vi "DAQ_Dyn Dig Gen Initialize.vi"(0 "Physical Channels":tag, 7 "Global Channels":refnum<k21>, 11 "error in":errorcluster) -> (4 "DAQmx Task Out":refnum<k21>, 15 "error out":errorcluster)   [LabVIEW 2021, in "DAQ_Dynamic Digital Pattern Generation.lvlib"]
doc: "Initialize Digital output channels and obtains a DAQmx task\n\nProvide either Physical channel or Global Channel\nIf both Physical and Global channels are provided, Global Channels will take precedence\n\nNote: This Library supports both <B>Port and Digital lines</B> from a single module to generate dynamic digital patterns. But <B>Multi-module</B> support is <B>not applicable</B> on this library and throws errors."
uses:
  DAQ_Dynamic Digital Pattern Generation.lvlib
  <vilib>/DAQmx/create/channels.llb/DAQmx Create Channel (DO-Digital Output).vi
panel:
  # "Inputs"
  # "Outputs"
  # "Overview:\nThis VI initializes Digital output channels for Dynamic digital pattern generation and provides the DAQmx Task Out\n\nHardware Requirement: A compatible PXI, PCIe, USB, cDAQ or Testscale device\n\nSoftware Requirement: NI DAQmx 2022Q4 or later\n\nInstructions:\n1. Enter physical channel in which Dynamic Digital Pattern Generation has to be done in Physical Channels control. (Or) Enter Global channels to use it instead of initiating a new task. User must configure only one input. If both are provided, Global Channels will take precedence.\n2. Get the Dynamic digital pattern generation task from DAQmx Task Out which stores the reference to the virtual digital output channels.\n\nNotes: \n1. User can use the DAQmx Task on other VI in this library to configure and initiate dynamic digital pattern generation task.\n2. This Library supports both Port and Digital lines from a single module to generate dynamic digital patterns. But Multi-module support is not applicable on this library and throws errors."
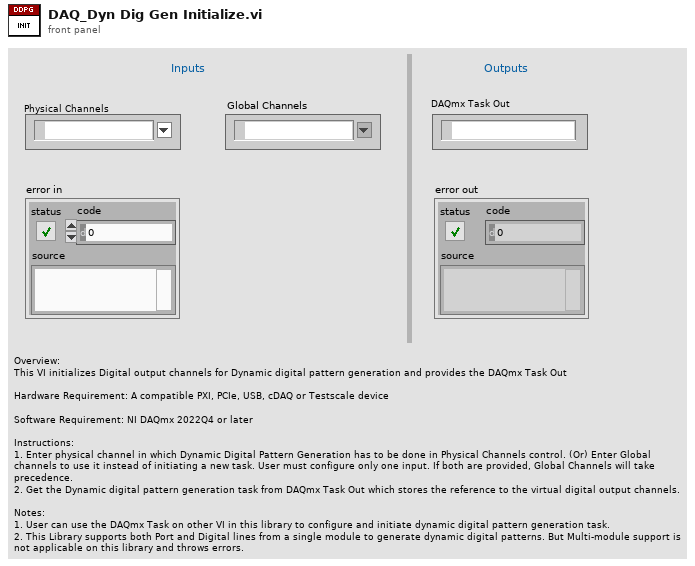
[diagram p1: front panel]
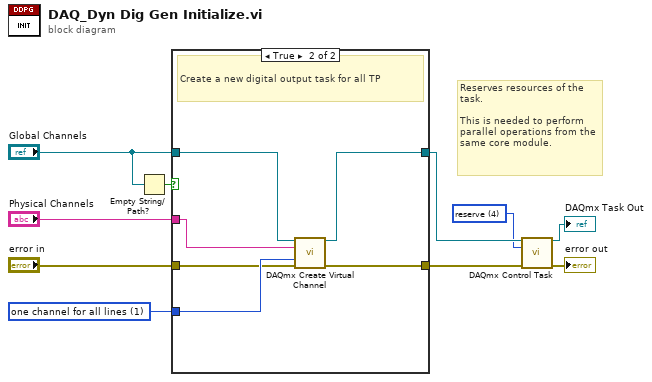
[diagram p0: block diagram]
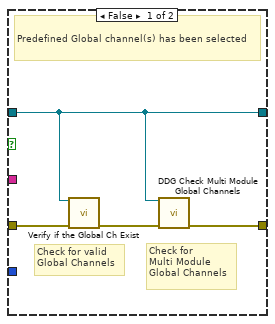
[diagram p2: hidden frame]
diagram:
  w1 = 4 items=["verify"=2, "reserve"=4, "commit"=3, "unreserve"=5, "abort"=6] ("action")
  w5 = 1 items=["one channel for each line", "one channel for all lines"] ("line grouping")
  # "Reserves resources of the task.\n\nThis is needed to perform parallel operations from the same core module."
  n1 = Empty String/Path?(string/path="Global Channels") -> (empty?=w7:bool)
  n2 = case shown="True" w7 {
    tunnel: "Physical Channels" -> [_ w15]
    tunnel: "Global Channels" -> [w11 w20]
    tunnel: [w11 w19] -> w3
    tunnel: "error in" -> [w13 w16]
    tunnel: [w14 w18] -> w10
    tunnel: w5 -> [_ w17]
    frame False {
      # "Check for \nMulti Module\nGlobal Channels"
      # "Check for valid \nGlobal Channels"
      # "Predefined Global channel(s) has been selected"
      n3 = call "Verify if the Global Ch Exist.vi"("Global Channels"=w11, "error in (no error)"=w13) -> ("error out"=w12:errorcluster)  [unwired: 13 in]
      n4 = call "DDG Check Multi Module Global Channels.vi"("Global Channel In"=w11, "error in (no error)"=w12) -> ("error out"=w14:errorcluster)  [unwired: 12 in, 1 out]
    }
    frame True {
      # "Create a new digital output task for all TP"
      n5 = call-poly <vilib>:"DAQmx Create Virtual Channel.vi"("task in"=w20, "lines"=w15, "line grouping"=w17, "error in"=w16) -> ("task out"=w19:refnum<k21>, "error out"=w18:errorcluster)  [unwired: 10 in]
    }
  }
  n6 = call <vilib>:"DAQmx Control Task.vi"("task/channels in"=w3, "action"=w1, "error in"=w10) -> ("task out"=→"DAQmx Task Out":refnum<k21>, "error out"=→"error out":errorcluster)  [unwired: 11 in]
